vi "Timeout dialoge Abbort.vi"(0 "Enable":bool=TRUE, 2 "Message to Display":string="Realy abbort measurement?", 3 "timeout[ms]":u32=5000, 5 "error in (no error)":errorcluster) -> (18 "Yes":bool, 19 "error out":errorcluster)   [LabVIEW 2021, in "MatS Libs.lvlib"]
doc: "Displays a standard dialog box that prompts users to enter information, such as a user name and password.\n--------------------\n\nThis Express VI is configured as follows:\n\nMessage to Display to the User:\nThe inputs are:"
uses:
  <userlib>/MatS Libs/MatS Libs.lvlib
panel:
  out "String":string
  in  "Cancel":bool
  in  "OK2":bool
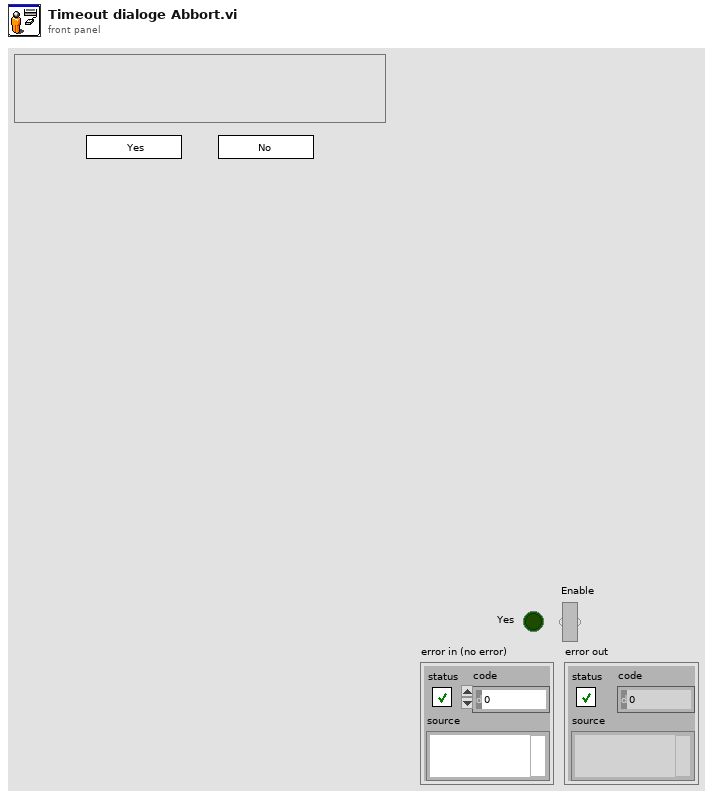
[diagram p1: front panel]
types:
  T1 = cluster{"Input Name":string, "Input Data Type":i32}[]
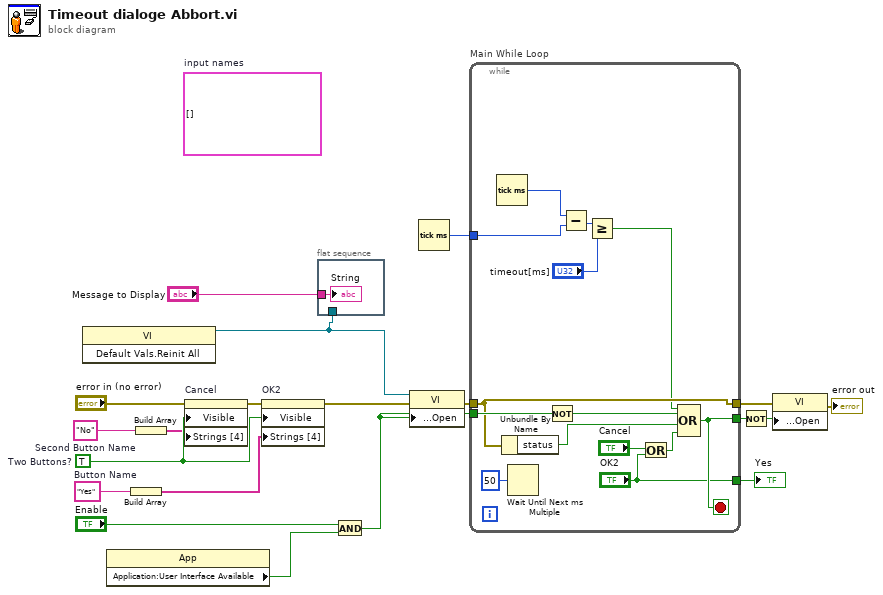
[diagram p0: block diagram]
diagram:
  (unwired) T1 []  # input names
  w14 = "No"  # Second Button Name
  w12 = "Yes"  # Button Name
  w20 = TRUE  # Two Buttons?
  n1 = invoke class="VI" method="Default Vals.Reinit All"() -> (reference out=w1:refnum<vi>)  [unwired: 3 in, 2 out]
  n2 = property class="App"() -> ("Application:User Interface Available"=w5:bool)  [unwired: 2 in, 2 out]
  n3 = Build Array(w12) -> (w13:string[])
  n4 = Build Array(w14) -> (w15:string[])
  n5 = property on="Cancel" class="Bool"(error in="error in (no error)", "Visible"=w20, "Strings [4]"=w15) -> (error out=w18:errorcluster)  [unwired: 1 in, 1 out]
  n6 = property on="OK2" class="Bool"(error in=w18, "Visible"=w20, "Strings [4]"=w13) -> (error out=w4:errorcluster)  [unwired: 1 in, 1 out]
  n7 = flat-sequence {
    tunnel: "Message to Display" -> [w21]
    tunnel: w1 -> [_]
    frame #0 {
      "String" <- w21
    }
  }
  n8 = And(x="Enable", y=w5) -> (x .and. y?=w6:bool)
  n9 = property class="VI"(reference=w1, error in=w4, "Front Panel Window:Open"=w6) -> (error out=w11:errorcluster)  [unwired: 1 out]
  n10 = Tick Count (ms)() -> (millisecond timer value=w3:u32)
  n11 = while "Main While Loop" {
    tunnel: ["OK2"] -> w19
    tunnel: w6 -> [w33]
    tunnel: [w31] -> w16
    tunnel: w11 -> [w30]
    tunnel: [w30] -> w9
    tunnel: w3 -> [w26]
    stop <- w31 stop-if-true
    n12 = Tick Count (ms)() -> (millisecond timer value=w27:u32)
    n13 = Unbundle By Name(w30) -> ("status"=w28:bool)
    n14 = Wait Until Next ms Multiple(millisecond multiple=u32 50) -> ()  [unwired: 1 out]
    n15 = Not(x=w33) -> (.not. x?=w32:bool)
    n16 = Subtract(x=w27, y=w26) -> (x-y=w25:u32)
    n17 = Greater Or Equal?(x=w25, y="timeout[ms]") -> (x >= y?=w23:bool)
    n18 = Or(x="Cancel", y="OK2") -> (x .or. y?=w29:bool)
    n19 = Compound Arithmetic op=OR(w23, w32, w28, w29) -> (w31:bool)
  }
  "Yes" <- w19
  n20 = Not(x=w16) -> (.not. x?=w17:bool)
  n21 = property class="VI"(error in=w9, "Front Panel Window:Open"=w17) -> (error out=→"error out":errorcluster)  [unwired: 1 in, 1 out]
